vi "Set PID Paras.vi"(8 "error in (no error)":errorcluster, 10 "PID Paras":T1={"Output Range(deg/s)"={"output high"=720.0, "output low"=-720.0}, "PID gains"={"proportional gain (Kc)"=6.5, "integral time (Ti, min)"=0.0075, "derivative time (Td, min)"=0.0005}} {"PID gains"."derivative time (Td, min)" format="%.4f"; "PID gains"."integral time (Ti, min)" format="%.4f"; "PID gains"."proportional gain (Kc)" format="%.4f"; "Output Range(deg/s)"."output low" format="%.2f"; "Output Range(deg/s)"."output high" format="%.2f"}, 11 "SGDV_Ctrl_Class in":refnum<class "SGDV_Ctrl_Class.lvclass">) -> (0 "error out":errorcluster, 3 "SGDV_Ctrl_Class out":refnum<class "SGDV_Ctrl_Class.lvclass">)   [LabVIEW 2013, in "SGDV_Ctrl_v13_lib.lvlib" / "SGDV_Ctrl_Class.lvclass"]
uses:
  SGDV_Ctrl_Class.lvclass
  Controls and General VIs/PID Paras.ctl
  SGDV_Ctrl_Class.lvclass/SGDV_Ctrl_Class.ctl
  SGDV_Ctrl_v13_lib.lvlib
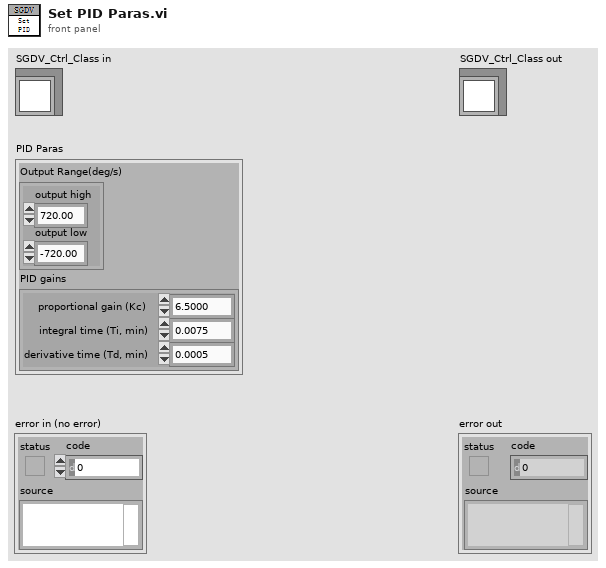
[diagram p1: front panel]
types:
  T1 = typedef "SGDV_Ctrl_v13_lib.lvlib/PID Paras.ctl" = cluster{"Output Range(deg/s)":cluster{"output high":dbl, "output low":dbl}, "PID gains":cluster{"proportional gain (Kc)":dbl, "integral time (Ti, min)":dbl, "derivative time (Td, min)":dbl}}
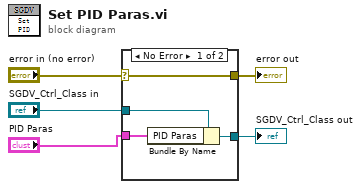
[diagram p0: block diagram]
diagram:
  n1 = case shown="No Error" "error in (no error)" {
    selector: "error in (no error)" -> [w9 w10]
    tunnel: [w9 w10] -> w4
    tunnel: [w7 w11] -> w2
    tunnel: "SGDV_Ctrl_Class in" -> [w8 w11]
    tunnel: "PID Paras" -> [w6 _]
    frame No Error {
      n2 = Bundle By Name(cluster=w8, "PID Paras"=w6) -> (w7:refnum<class "SGDV_Ctrl_Class.lvclass">)
    }
    frame Error {
    }
  }
  "error out" <- w4
  "SGDV_Ctrl_Class out" <- w2
